vi "GetSweepInfoByChannel.vi"(10 "AssetNodes":T1[](array[typedef]), 11 "AssetNodeId":string) -> (3 "sweeps":T12[](array[typedef]))   [LabVIEW 2017, in "EmsaAnalysis.lvlib"]
uses:
  <vilib>/addons/InsightCM/Devices/Shared/Emsa/EmsaAnalysis/EmsaAnalysis.lvlib
  <vilib>/addons/InsightCM/Devices/Shared/Emsa/EmsaAnalysis/controls/sweepInfo.ctl
  <vilib>/addons/InsightCM/MessageBus/Base/controls/AssetNode.ctl
  <vilib>/addons/InsightCM/MessageBus/Base/controls/AssetState.ctl
  <vilib>/addons/InsightCM/MessageBus/Base/controls/KeyValuePair.ctl
  <vilib>/addons/InsightCM/MessageBus/Base/controls/OperatingState.ctl
  <vilib>/addons/InsightCM/MessageBus/Base/controls/Trigger.ctl
  <vilib>/addons/InsightCM/MessageBus/Base/controls/Condition.ctl
  <vilib>/addons/InsightCM/MessageBus/Base/controls/Metric.ctl
  <vilib>/addons/InsightCM/MessageBus/Base/controls/TrendAlarmRule.ctl
  <vilib>/addons/InsightCM/MessageBus/Base/controls/TrendAlarmLevel.ctl
  <vilib>/addons/InsightCM/MessageBus/Base/controls/AlarmAction.ctl
  <vilib>/addons/InsightCM/MessageBus/Base/controls/AssetNodeReference.ctl
  <vilib>/addons/InsightCM/Utilities/PropertyHelpers/PropertyHelpers.lvlib
  <vilib>/addons/InsightCM/Utilities/DeviceModelHelpers/DeviceModelHelpers.lvlib
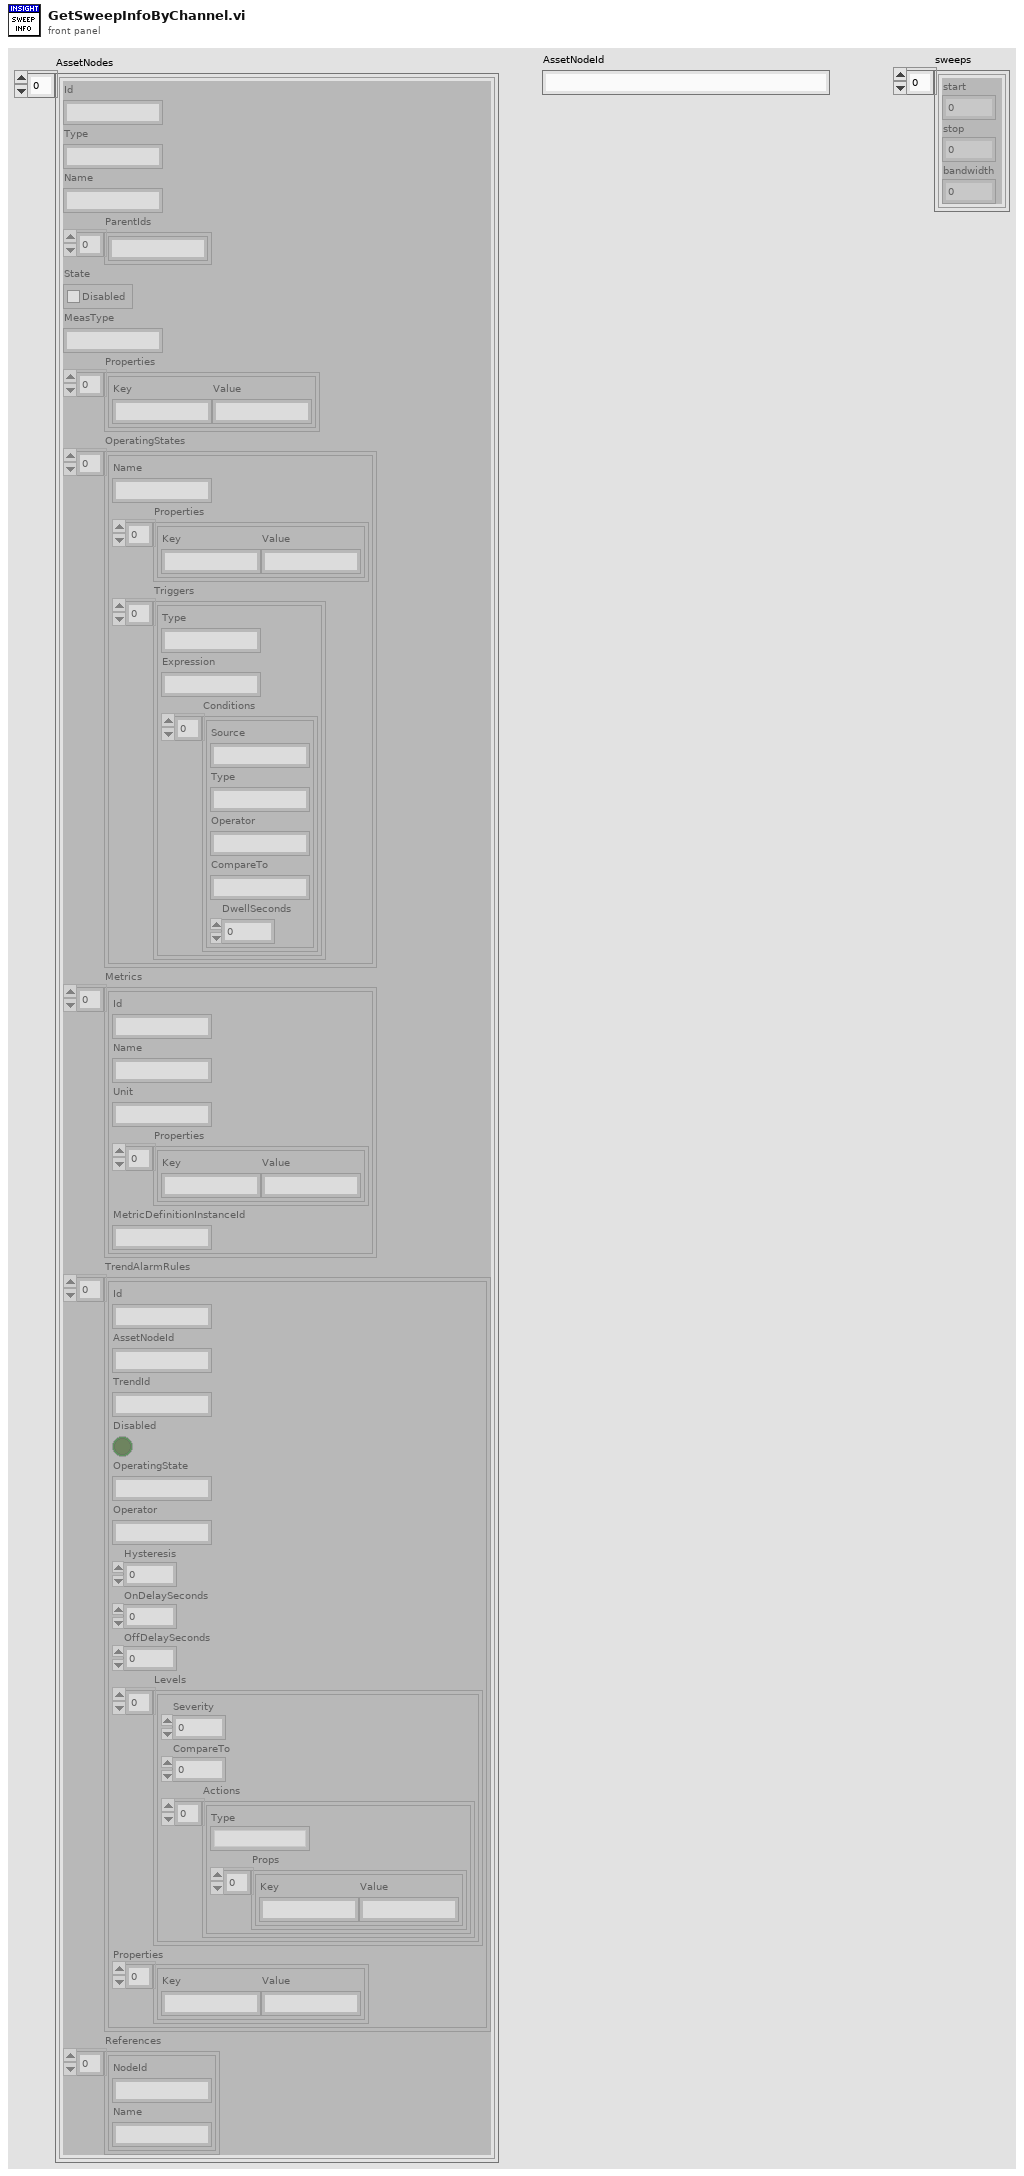
[diagram p1: front panel]
types:
  T1 = typedef "AssetNode.ctl" = cluster{"Id":string, "Type":string, "Name":string, "ParentIds":string[], "State":T2, "MeasType":string, "Properties":T3[], "OperatingStates":T4[], "Metrics":T7[], "TrendAlarmRules":T8[], "References":T11[]}
  T2 = typedef "AssetState.ctl" = cluster{"Disabled":bool}
  T3 = typedef "KeyValuePair.ctl" = cluster{"Key":string, "Value":string}
  T4 = typedef "OperatingState.ctl" = cluster{"Name":string, "Properties":T3[], "Triggers":T5[]}
  T5 = typedef "Trigger.ctl" = cluster{"Type":string, "Expression":string, "Conditions":T6[]}
  T6 = typedef "Condition.ctl" = cluster{"Source":string, "Type":string, "Operator":string, "CompareTo":string, "DwellSeconds":dbl}
  T7 = typedef "Metric.ctl" = cluster{"Id":string, "Name":string, "Unit":string, "Properties":T3[], "MetricDefinitionInstanceId":string}
  T8 = typedef "TrendAlarmRule.ctl" = cluster{"Id":string, "AssetNodeId":string, "TrendId":string, "Disabled":bool, "OperatingState":string, "Operator":string, "Hysteresis":dbl, "OnDelaySeconds":dbl, "OffDelaySeconds":dbl, "Levels":T9[], "Properties":T3[]}
  T9 = typedef "TrendAlarmLevel.ctl" = cluster{"Severity":i32, "CompareTo":dbl, "Actions":T10[]}
  T10 = typedef "AlarmAction.ctl" = cluster{"Type":string, "Props":T3[]}
  T11 = typedef "AssetNodeReference.ctl" = cluster{"NodeId":string, "Name":string}
  T12 = typedef "EmsaAnalysis.lvlib/sweepInfo.ctl" = cluster{"start":dbl, "stop":dbl, "bandwidth":dbl}
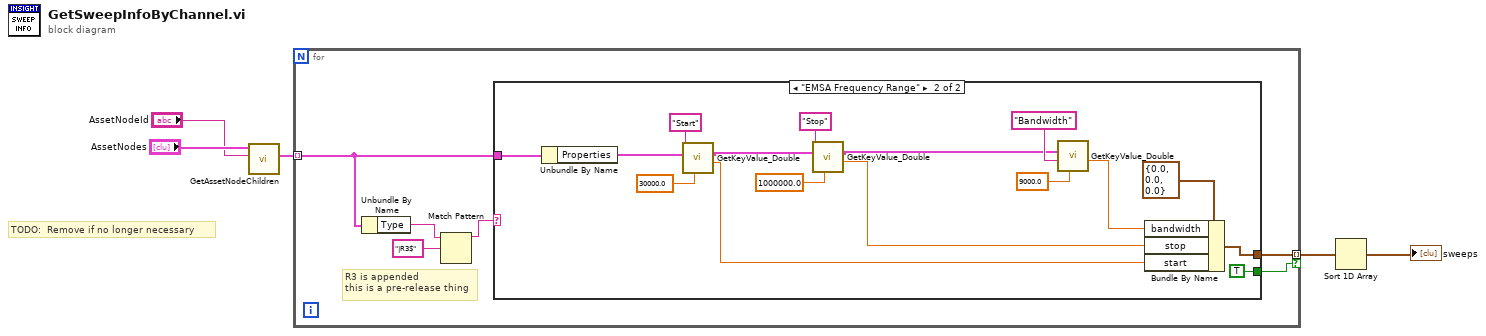
[diagram p0: block diagram]
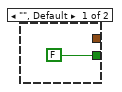
[diagram p2: hidden frame]
diagram:
  # "TODO:  Remove if no longer necessary"
  n1 = call <vilib>:"GetAssetNodeChildren.vi"("node id"="AssetNodeId", "nodes in"="AssetNodes") -> ("Children"=w3:T1[])  [unwired: 8 in, 1 out]
  n2 = for {
    tunnel: [w11] -> w1 mode=indexing if=w6
    tunnel: w3 -> [w10] mode=indexing
    # "R3 is appended\nthis is a pre-release thing"
    n3 = Unbundle By Name(w10) -> ("Type"=w8:string)
    n4 = Match Pattern(string=w8, regular expression="|R3$") -> (before substring=w7:string)  [unwired: 1 in, 3 out]
    n5 = case shown="\"EMSA Frequency Range\"" w7 {
      tunnel: [_ w18] -> w11
      tunnel: w10 -> [_ w17]
      tunnel: [FALSE TRUE] -> w6
      frame "", Default {
      }
      frame "EMSA Frequency Range" {
        n6 = Unbundle By Name(w17) -> ("Properties"=w16:T3[])
        n7 = call <vilib>:"GetKeyValue_Double.vi"("default"=30000.0, "key"="Start", "key value pairs"=w16) -> ("value"=w19:dbl, "key value pairs out"=w24:T3[])  [unwired: 6 in, 1 out]
        n8 = call <vilib>:"GetKeyValue_Double.vi"("default"=1000000.0, "key"="Stop", "key value pairs"=w24) -> ("value"=w20:dbl, "key value pairs out"=w13:T3[])  [unwired: 6 in, 1 out]
        n9 = call <vilib>:"GetKeyValue_Double.vi"("default"=9000.0, "key"="Bandwidth", "key value pairs"=w13) -> ("value"=w21:dbl)  [unwired: 6 in, 2 out]
        n10 = Bundle By Name(cluster=T12 {"start"=0.0, "stop"=0.0, "bandwidth"=0.0} ("sweep info"), "bandwidth"=w21, "stop"=w20, "start"=w19) -> (w18:T12)
      }
    }
  }
  n11 = Sort 1D Array(array=w1) -> (sorted array=→"sweeps":T12[])
